vi "DHE_SetTP.vi"(4 "Database RefNum in":T1, 6 "phys. unit":string, 7 "switches":string[](array[string]), 8 "error in (no error)":errorcluster, 9 "index in":i32, 10 "TP In":T2={"name"="", "type"="", "R_algor"=[], "board"="", "memory"="", "address"=0, "value"="", "Limits"={"upper"=0.0, "Lower"=0.0, "InRange"=FALSE, "nominal"=0.0}, "unit"="", "params"="", "permissions"="", "W_algor"=[], "description"="", "err_count"=0, "max_err"=3, "read"=FALSE, "lowrej"=0.0, "hirej"=0.0, "expupd"=FALSE} {"Limits"."nominal" format="%.2f"; "Limits"."Lower" format="%.2f"; "Limits"."upper" format="%.2f"}, 11 "refnum":i32) -> (0 "error out":errorcluster, 1 "In Range?":bool, 2 "response":string, 3 "refnum out":i32)   [LabVIEW 2016]
uses:
  DHE_TP.ctl
  DBSHAND/private/vis/DatabaseHand_RefNum.ctl
  DHE_TPLimits.ctl
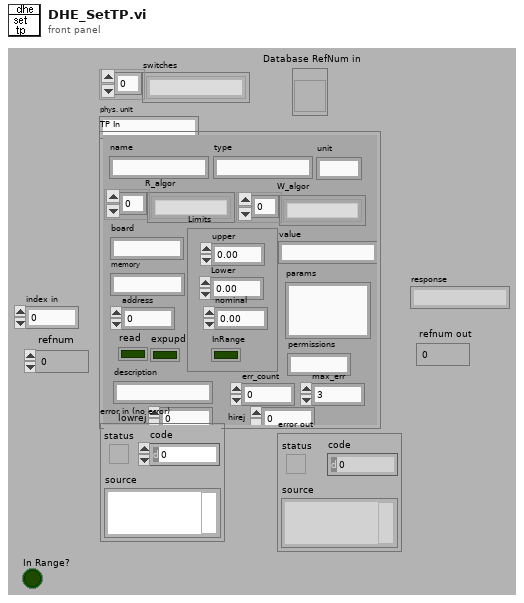
[diagram p1: front panel]
types:
  T1 = typedef "DatabaseHand_RefNum.ctl" = refnum<vi>
  T2 = typedef "DHE_TP.ctl" = cluster{"name":string, "type":string, "R_algor":string[], "board":string, "memory":string, "address":i32, "value":string, "Limits":T3, "unit":string, "params":string, "permissions":string, "W_algor":string[], "description":string, "err_count":i32, "max_err":i32, "read":bool, "lowrej":dbl, "hirej":dbl, "expupd":bool}
  T3 = typedef "DHE_TPLimits.ctl" = cluster{"upper":dbl, "Lower":dbl, "InRange":bool, "nominal":dbl}
  T4 = enum16{"READ FROM FILE", "GET ALL", "FIND BY NAME", "FIND BY TYPE", "SET VALUE", "CLEAN"}
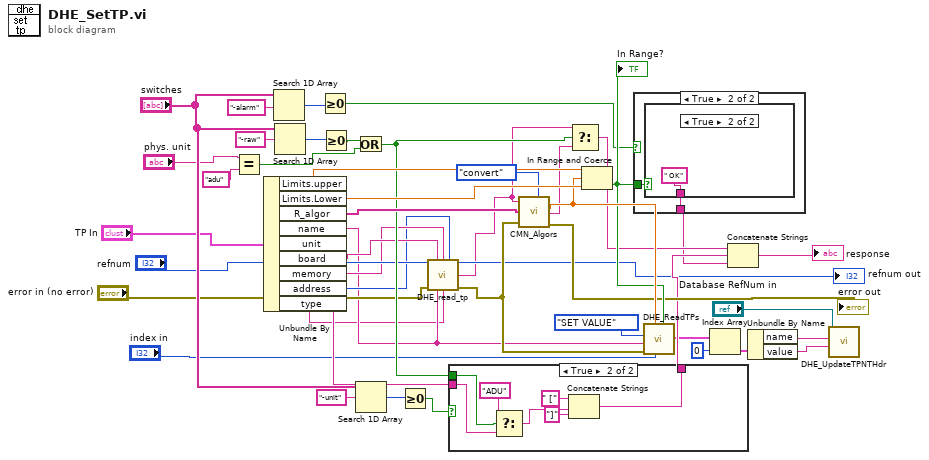
[diagram p0: block diagram]
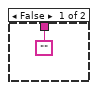
[diagram p2: hidden frame]
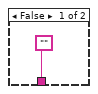
[diagram p3: hidden frame]
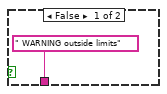
[diagram p4: hidden frame]
diagram:
  n1 = Equal?(x="phys. unit", y="adu") -> (x = y?=w23:bool)
  n2 = Unbundle By Name("TP In") -> ("Limits.upper"=w46:dbl, "Limits.Lower"=w45:dbl, "R_algor"=w36:string[], "name"=w5:string, "unit"=w27:string, "board"=w9:string, "memory"=w8:string, "address"=w7:i32, "type"=w4:string)
  n3 = Search 1D Array(1D array="switches", element="-alarm") -> (index of element=w32:i32)  [unwired: 1 out]
  n4 = Search 1D Array(1D array="switches", element="-raw") -> (index of element=w39:i32)  [unwired: 1 out]
  n5 = Greater Or Equal To 0?(x=w32) -> (x >= 0?=w31:bool)
  n6 = Greater Or Equal To 0?(x=w39) -> (x >= 0?=w26:bool)
  n7 = Or(x=w26, y=w23) -> (x .or. y?=w25:bool)
  n8 = Search 1D Array(1D array="switches", element="-unit") -> (index of element=w29:i32)  [unwired: 1 out]
  n9 = Greater Or Equal To 0?(x=w29) -> (x >= 0?=w28:bool)
  n10 = call "DHE_read_tp.vi"("fd"="refnum", "board"=w9, "memory"=w8, "address"=w7, "error in (no error)"="error in (no error)", "name"=w5, "type"=w4) -> ("fd out"=→"refnum out":i32, "return value"=w6:string, "error out"=w11:errorcluster)  [unwired: 6 out]
  n11 = case shown="True" w28 {
    tunnel: w27 -> [_ w51]
    tunnel: w25 -> [_ w52]
    tunnel: ["" w48] -> w22
    frame False {
    }
    frame True {
      n12 = Select(t="ADU", s=w52, f=w51) -> (s? t:f=w49:string)
      n13 = Concatenate Strings(" [" ("string"), w49, "]" ("string")) -> (w48:string)
    }
  }
  n14 = call "CMN_Algors.vi"("ValueIn"=w6, "algors"=w36, "error in (no error)"=w11, "action"=enum16{"convert", "read from file", "get"}."convert") -> ("Value out"=w42:sgl, "string value"=w38:string, "error out"=→"error out":errorcluster)  [unwired: 1 in, 3 out]
  n15 = Select(t=w6, s=w25, f=w38) -> (s? t:f=w37:string)
  n16 = In Range and Coerce(upper limit=w46, x=w42, lower limit=w45) -> (In Range?=w41:bool)  [unwired: 1 out]
  "In Range?" <- w41
  n17 = case shown="True" w31 {
    tunnel: ["" w57] -> w21
    tunnel: w41 -> [_ w56]
    frame False {
    }
    frame True {
      n18 = case shown="True" w56 {
        tunnel: [" WARNING outside limits" " OK"] -> w57
        frame False {
        }
        frame True {
        }
      }
    }
  }
  n19 = call "DHE_ReadTPs.vi"("inRange"=w41, "index in"="index in", "value"=w42, "error in (no error)"=w11, "argument"=w5, "action"=T4."SET VALUE") -> ("TPs"=w16:T2[])  [unwired: 1 in, 4 out]
  n20 = Index Array(array=w16, index=0) -> (element=w3:T2)
  n21 = Concatenate Strings(w37, w22, w21) -> (→"response":string)
  n22 = Unbundle By Name(w3) -> ("name"=w2:string, "value"=w1:string)
  n23 = call "DHE_UpdateTPNTHdr.vi"("TP value"=w1, "TP name"=w2, "Database RefNum in"="Database RefNum in") -> ()  [unwired: 1 in, 8 out]
